vi "Main.vi"(0 "Command":string) -> (4 "Response":string)   [LabVIEW 2020]
doc: "This VI gets in commands from user as SOURce and MEASure and the calls a subVI to write and get the values from the file to return and also logs this event with time"
panel:
  in  "Error in":errorcluster
  in  "Error":dbl=0.1
  out "Error out":errorcluster
  # "This VI give commands from user to another VI to store the data and then \nretrives it based on the command input"
  # "Command Input:\n1. Write:  SOURce:VOLTage/CURRent:DC ?\n2. Read:   MEASure:VOLTage/CURRent:DC"
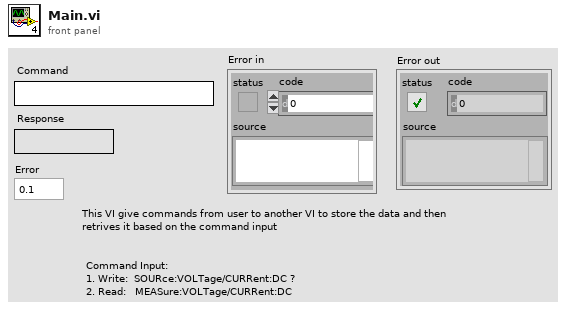
[diagram p1: front panel]
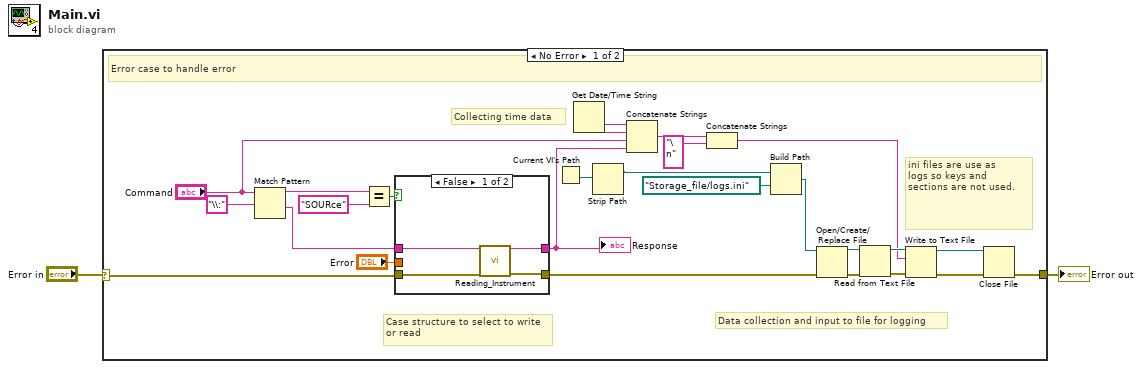
[diagram p0: block diagram]
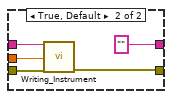
[diagram p2: hidden frame]
diagram:
  n1 = case shown="No Error" "Error in" {
    selector: "Error in" -> [w3 w38]
    tunnel: [w14 w38] -> w2
    frame No Error {
      # "Collecting time data"
      # "ini files are use as\nlogs so keys and \nsections are not used."
      # "Case structure to select to write\nor read"
      # "Data collection and input to file for logging"
      # "Error case to handle error"
      n2 = Match Pattern(string="Command", regular expression="\\:") -> (before substring=w27:string, after substring=w24:string)  [unwired: 1 in, 2 out]
      n3 = Equal?(x=w27, y="SOURce") -> (x = y?=w25:bool)
      n4 = case shown="False" w25 {
        tunnel: w24 -> [w32 w34]
        tunnel: [w31 "" ("String 3")] -> w15
        tunnel: "Error" -> [_ w33]
        tunnel: [w29 w35] -> w4
        tunnel: w3 -> [w30 w36]
        frame False {
          n5 = call "Reading_Instrument.vi"("Read String"=w32, "error in"=w30) -> ("Readed Data"=w31:string, "error out"=w29:errorcluster)  [unwired: 12 in]
        }
        frame True, Default {
          n6 = call "Writing_Instrument.vi"("Write String"=w34, "Error"=w33, "error in"=w36) -> ("error out"=w35:errorcluster)  [unwired: 12 in]
        }
      }
      "Response" <- w15
      n7 = Current VI's Path() -> (path=w21:path)
      n8 = Get Date/Time String() -> (date string=w18:string, time string=w17:string)  [unwired: 3 in]
      n9 = Strip Path(path=w21) -> (stripped path=w13:path)  [unwired: 1 out]
      n10 = Concatenate Strings(w18, w17, "Command", w15) -> (w8:string)
      n11 = Concatenate Strings(w8, "\n" ("string")) -> (w6:string)
      n12 = Build Path(base path=w13, name or relative path=path "Storage_file/logs.ini") -> (appended path=w19:path)
      n13 = Open/Create/Replace File(file path (use dialog)=w19, error in=w4) -> (refnum out=w10:refnum<file>, error out=w12:errorcluster)  [unwired: 4 in, 1 out]
      n14 = Read from Text File(file (use dialog)=w10, error in=w12) -> (refnum out=w9:refnum<file>, error out=w11:errorcluster)  [unwired: 2 in, 2 out]
      n15 = Write to Text File(file (use dialog)=w9, text=w6, error in=w11) -> (refnum out=w22:refnum<file>, error out=w23:errorcluster)  [unwired: 1 in, 1 out]
      n16 = Close File(refnum=w22, error in=w23) -> (error out=w14:errorcluster)  [unwired: 1 out]
    }
    frame Error {
    }
  }
  "Error out" <- w2
